vi "SensorFileHeader.vi"() -> (0 "Header\nOut":string[](array[string]))   [LabVIEW 2020]
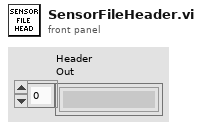
[diagram p1: front panel]
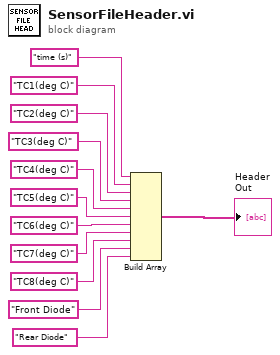
[diagram p0: block diagram]
diagram:
  n1 = Build Array("time (s)", "TC1(deg C)", "TC2(deg C)", "TC3(deg C)", "TC4(deg C)", "TC5(deg C)", "TC6(deg C)", "TC7(deg C)", "TC8(deg C)", "Front Diode", "Rear Diode") -> (→"Header\nOut":string[])
